vi "stop.vi"(7 "emergency_stop":string, 8 "LabVIEW Web Service Request":refnum<class "Web Request.lvclass">, 24 "end_stage":string) -> ()   [LabVIEW 2020]
uses:
  <vilib>/wsapi/Web Request.lvclass
  Global 1.vi
panel:
  # "Use the Web Service Request input terminal to call the VIs on the Web Services palette. Do not remove it from the connector pane unless you don't need access to the palette."
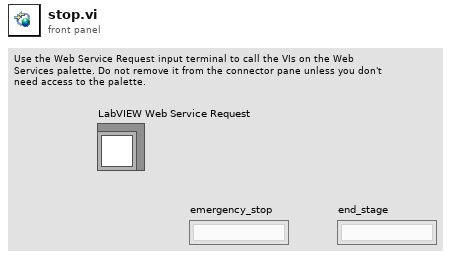
[diagram p1: front panel]
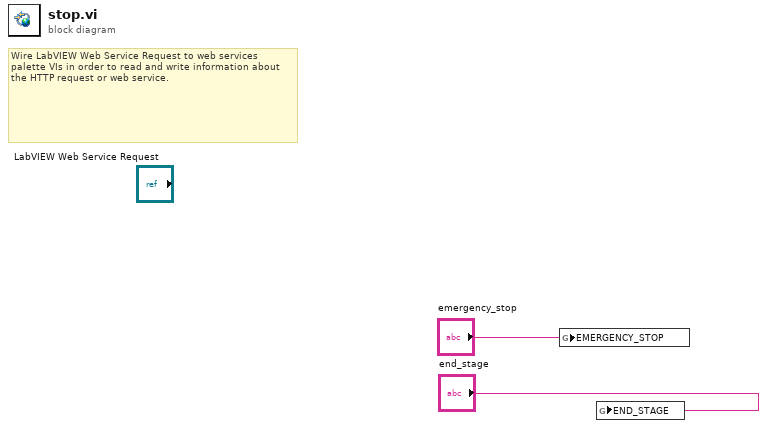
[diagram p0: block diagram]
diagram:
  # "Wire LabVIEW Web Service Request to web services palette VIs in order to read and write information about the HTTP request or web service."
  n1 = global write "Global 1.vi" "EMERGENCY_STOP"("emergency_stop") -> ()
  n2 = global write "Global 1.vi" "END_STAGE"("end_stage") -> ()
